vi "Process Incoming Messages.vi"(8 "error in":errorcluster, 10 "CAN frame":T14 {"payload" format="%x"; "timestamp" format="%<%.7X\n%x>T"; "type" items=["CAN Data"=0, "CAN Remote"=1, "CAN Bus Error"=2, "J1939 Data"=192, "Delay"=224, "Log Trigger"=225, "Start Trigger"=226]; "identifier" format="%x"}, 11 "internal data":T1={"J1939 XNET Settings"={"XNET Database"="", "XNET Cluster"="", "CAN port"="", "Baud rate [Bd]"=0, "J1939 Network Address"=0, "Name"=0, "Termination"=0}, "j1939 queues"={"Processed Outgoing"=refnum, "Process Outgoing"=refnum, "stop notifier"=refnum, "error queue"=refnum, "active dtc"=refnum, "processed inc"=refnum}, "fgv references"={"BAM Buffer"=refnum, "CM Buffer"=refnum, "CM Gen"=refnum, "BAM Gen"=refnum, "Address Claims"=refnum, "RQST"=refnum, "scaling lut"=refnum, "data lut"=refnum, "cyclic scheduler"=refnum}, "frame in"="", "frame out"="", "timing"={"tb to j1939 queue timeout"=100, "j1939 to tb queue timeout"=100, "dtc loop period (ms)"=100, "CAN in loop period (ms)"=100, "process incoming queue timeout (ms)"=100, "Outgoing Write Decimation"=0, "process outgoing loop rate (ms)"=0, "periodic outgoing queue timeout (ms)"=10, "CAN out queue timeout (ms)"=100}}) -> (0 "error out":errorcluster)   [LabVIEW 2013, in "J1939.lvlib"]
uses:
  J1939.lvlib
  <vilib>/xnet/xnet.llb/XNET Frame CAN.ctl
  <vilib>/xnet/xnet.llb/XNET Frame Type CAN.ctl
  API Types/Internal Data.ctl
  API Types/XNET Settings.ctl
  API Types/Setup Information Cluster.ctl
  API Types/CAN Outgoing Message Cluster.ctl
  API Types/Convert DTCs Cluster.ctl
  TP/TP List References.ctl
  BAM/BAM Buffer Connections List_Ref.ctl
  Connection Mode/Connection Mode Generation Connection Ref.ctl
  BAM/BAM Generation Connections List_Ref.ctl
  LUTs/J1939 Address Table Reference.ctl
  RQST/RQST Lookup Table Reference.ctl
  LUTs/J1939 Conversion Lookup Table Reference.ctl
  LUTs/J1939 Data Lookup Table Reference.ctl
  LUTs/Cyclic Frame Scheduler Lut Reference.ctl
  Configuration/TypeDefs/timing configuration.ctl
  Parse Message Type.vi
  RQST/RQST Lookup Table Act.vi
  Frame Conversion/Common Conversions.vi
  Frame Conversion/Convert CAN Arb ID to J1939 ID.vi
  Frame Conversion/Convert J1939 ID to CAN Arb ID.vi
  Frame Conversion/Convert CAN Data (U32) to U8.vi
  Convert Signals to Frame by ID.vi
  Common Messages/J1939 Common Messages.vi
  Common Messages/J1939 Message Acknowledgement.vi
  BAM/BAM Buffer.vi
  Buffer Connections List_Actions.vi
  TP/TP Buffer Search for Connection (No PGN).vi
  TP/TP Buffer Add New Data Packet to Connection.vi
  TP/TP Buffer Convert Connection Info to CAN Frame.vi
  TP/TP Buffer Create New TP Connection.vi
  Connection Mode/Connnection Mode Buffer.vi
  Common Messages/J1939 Message TP.CM EndofMsgACK.vi
  Common Messages/J1939 Message TP.CM CTS.vi
  Common Messages/J1939 Message TP.Conn Abort.vi
  Connection Mode/Connection Mode Generation.vi
  Connection Mode/Connection Mode Generation Connections List_Actions.vi
  Connection Mode/Connection Mode Generation Search for Connection (Remote Message).vi
  TP/TP Buffer Search for Connection.vi
  Connection Mode/Connection Mode Generation CTS Received.vi
  LUTs/J1939 Network Address Lookup Table.vi
  Conversion Lookup Table Get Conversion Parameter.vi
  LUTs/J1939 Data Lookup Table Get Signals (Range).vi
  Frame Conversion/Convert PGN + SA to J1939 ID.vi
  <vilib>/xnet/xnet.llb/XNET Convert.vi
  <vilib>/xnet/xnet.llb/XNET Convert (Signal to Frame Raw).vi
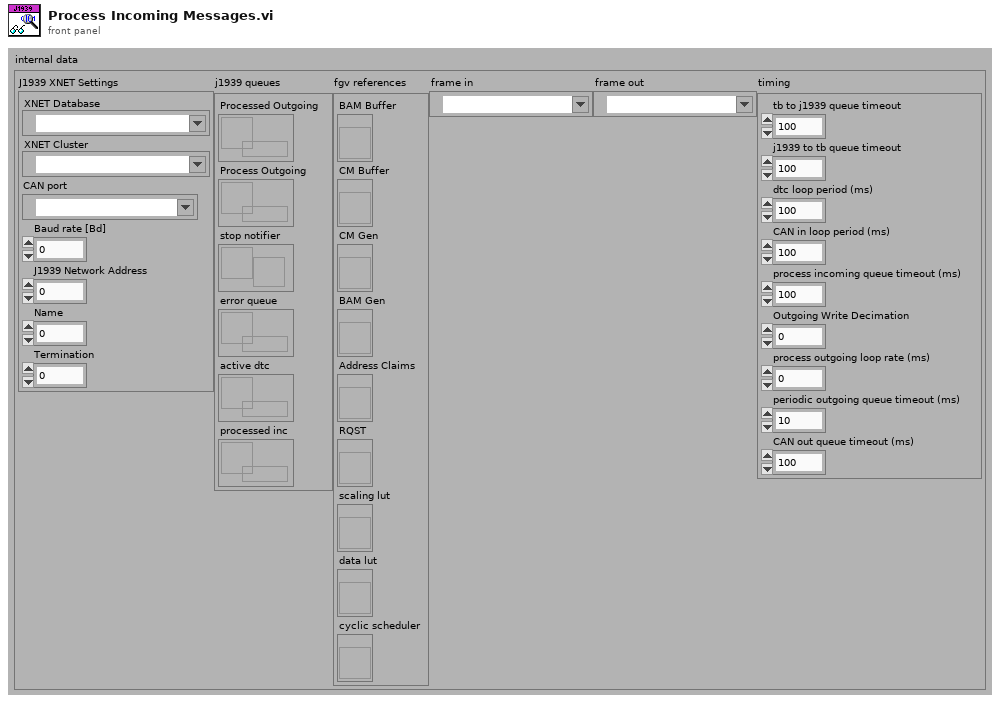
[diagram p1: front panel]
types:
  T1 = typedef "J1939.lvlib/Internal Data.ctl" = cluster{"J1939 XNET Settings":T2, "j1939 queues":T3, "fgv references":T4, "frame in":refnum<k21>, "frame out":refnum<k21>, "timing":T13}
  T2 = typedef "J1939.lvlib/XNET settings.ctl" = cluster{"XNET Database":refnum<k21>, "XNET Cluster":refnum<k21>, "CAN port":refnum<k21>, "Baud rate [Bd]":u32, "J1939 Network Address":u8, "Name":u64, "Termination":u32}
  T3 = typedef "J1939.lvlib/Setup Information Cluster.ctl" = cluster{"Processed Outgoing":refnum<queue>, "Process Outgoing":refnum<queue>, "stop notifier":refnum<notifier>, "error queue":refnum<queue>, "active dtc":refnum<queue>, "processed inc":refnum<queue>}
  T4 = typedef "J1939.lvlib/TP List References.ctl" = cluster{"BAM Buffer":T5, "CM Buffer":T5, "CM Gen":T6, "BAM Gen":T7, "Address Claims":T8, "RQST":T9, "scaling lut":T10, "data lut":T11, "cyclic scheduler":T12}
  T5 = typedef "J1939.lvlib/BAM Buffer Connections List_Ref.ctl" = refnum<vi>
  T6 = typedef "J1939.lvlib/Connection Mode Generation Connection Ref.ctl" = refnum<vi>
  T7 = typedef "J1939.lvlib/BAM Generation Connections List_Ref.ctl" = refnum<vi>
  T8 = typedef "J1939.lvlib/J1939 Address Table Reference.ctl" = refnum<vi>
  T9 = typedef "J1939.lvlib/RQST Lookup Table Reference.ctl" = refnum<vi>
  T10 = typedef "J1939.lvlib/J1939 Conversion Lookup Table Reference.ctl" = refnum<vi>
  T11 = typedef "J1939.lvlib/J1939 Data Lookup Table Reference.ctl" = refnum<vi>
  T12 = typedef "J1939.lvlib/cyclic frame scheduler lut reference.ctl" = refnum<vi>
  T13 = typedef "J1939.lvlib/timing configuration.ctl" = cluster{"tb to j1939 queue timeout":i32, "j1939 to tb queue timeout":i32, "dtc loop period (ms)":i32, "CAN in loop period (ms)":i32, "process incoming queue timeout (ms)":i32, "Outgoing Write Decimation":u32, "process outgoing loop rate (ms)":i32, "periodic outgoing queue timeout (ms)":i32, "CAN out queue timeout (ms)":i32}
  T14 = typedef "XNET Frame CAN.ctl" = cluster{"timestamp":timestamp, "payload":u8[], "identifier":u32, "type":T15, "extended?":bool, "echo?":bool}
  T15 = typedef "XNET Frame Type CAN.ctl" = u8
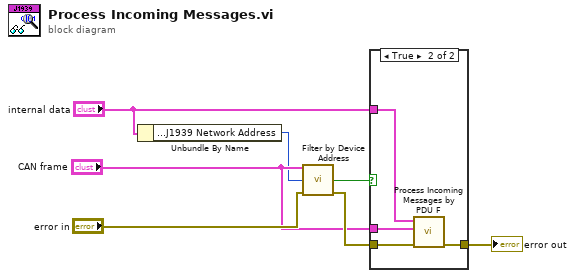
[diagram p0: block diagram]
diagram:
  n1 = Unbundle By Name("internal data") -> ("J1939 XNET Settings.J1939 Network Address"=w2:u8)
  n2 = call "Filter by Device Address.vi"("CAN Frame"="CAN frame", "Current Device Address"=w2, "error in"="error in") -> ("Pass Through"=w6:bool, "error out"=w5:errorcluster)  [unwired: 11 out]
  n3 = case shown="True" w6 {
    tunnel: [w8 w12] -> w4
    tunnel: w5 -> [w8 w11]
    tunnel: "CAN frame" -> [_ w9]
    tunnel: "internal data" -> [_ w10]
    frame False {
    }
    frame True {
      n4 = call "Process Incoming Messages by PDU F.vi"("error in"=w11, "CAN Frame"=w9, "internal data"=w10) -> ("error out"=w12:errorcluster)  [unwired: 8 in]
    }
  }
  "error out" <- w4
